vi "Initialize Sim youBot Gripper.vi"(8 "error in (no error)":errorcluster, 10 "arm index":i32, 11 "robot ID":string) -> (0 "error out":errorcluster, 3 "simulated KUKA youBot gripper out":refnum<class "NI_Robotics_KUKA youBot Gripper_Sim.lvclass">)   [LabVIEW 2017, in "NI_Robotics_KUKA youBot Host.lvlib" / "NI_Robotics_KUKA youBot Gripper_Sim.lvclass"]
uses:
  <vilib>/robotics/KUKA youBot/Basic Device/Gripper Sim/NI_Robotics_KUKA youBot Gripper_Sim.lvclass
  c:/Program Files (x86)/National Instruments/LabVIEW 2017/vi.lib/robotics/KUKA youBot/Basic Device/Gripper/NI_Robotics_KUKA youBot Gripper.lvclass
  <vilib>/robotics/Simulator/Engine/ctl/DeviceID.ctl
  <vilib>/robotics/KUKA youBot/Motor/Gripper Motor Sim/NI_Robotics_KUKA youBot Gripper Motor_Sim.lvclass
  c:/Program Files (x86)/National Instruments/LabVIEW 2017/vi.lib/robotics/KUKA youBot/Motor/Gripper Motor/NI_Robotics_KUKA youBot Gripper Motor.lvclass
  <vilib>/robotics/Simulator/NI_Robotics_Simulator.lvlib
  <vilib>/robotics/KUKA youBot/Basic Device/Gripper/NI_Robotics_KUKA youBot Gripper.lvclass
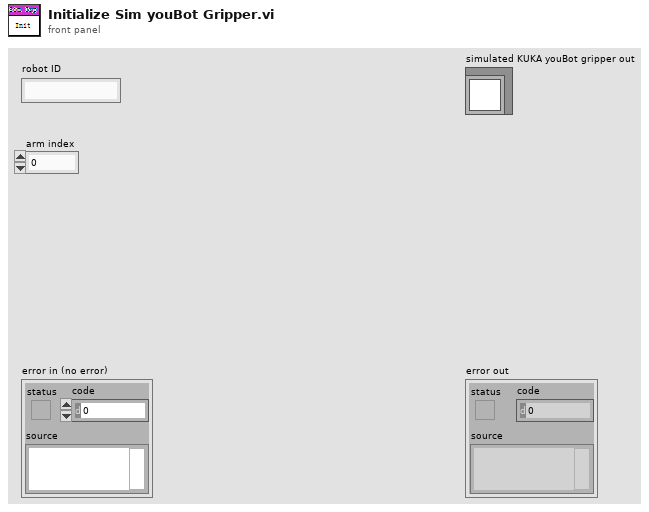
[diagram p1: front panel]
types:
  T1 = typedef "NI_Robotics_Simulator.lvlib/DeviceID.ctl" = cluster{"robot ID":string, "sensor/actuator ID":string}
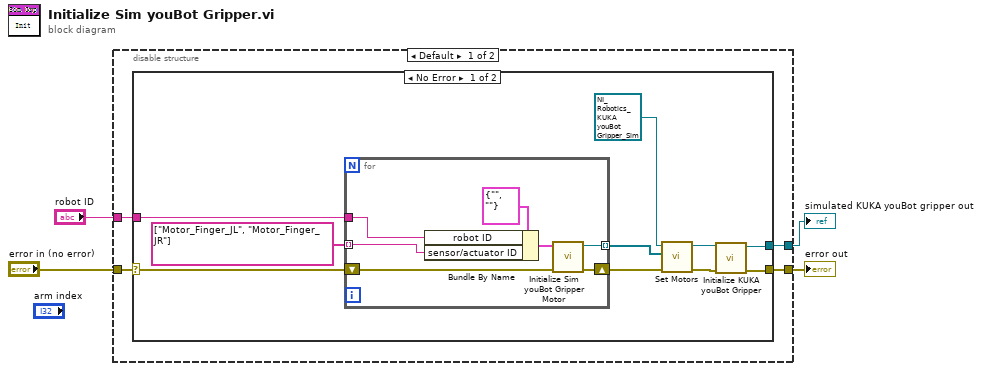
[diagram p0: block diagram]
diagram:
  n1 = disable-structure shown="Default" {
    disable-tunnel: "error in (no error)" -> [w8 _]
    disable-tunnel: [w7 _] -> w3
    disable-tunnel: "robot ID" -> [w6 _]
    disable-tunnel: [w5 _] -> w1
    frame condition #0 (active) {
      n2 = case shown="No Error" w8 {
        selector: w8 -> [w16 w26]
        tunnel: [w10 w26] -> w7
        tunnel: w6 -> [w18 _]
        tunnel: [w9 _] -> w5
        frame No Error {
          n3 = for {
            tunnel: w18 -> [w24]
            tunnel: string[] ["Motor_Finger_JL", "Motor_Finger_JR"] -> [w23] mode=indexing
            shift-right: [w20] -> w14
            shift-left: w16 -> [w21]
            tunnel: [w19] -> w13 mode=indexing
            n4 = Bundle By Name(cluster=T1 {"robot ID"="", "sensor/actuator ID"=""} ("device ID"), "robot ID"=w24, "sensor/actuator ID"=w23) -> (w22:T1)
            n5 = call <vilib>:"Initialize Sim youBot Gripper Motor.vi"("error in (no error)"=w21, "device ID"=w22) -> ("error out"=w20:errorcluster, "simulated KUKA youBot gripper motor out"=w19:refnum<class "NI_Robotics_KUKA youBot Gripper Motor_Sim.lvclass">)  [unwired: 8 in]
          }
          n6 = call-dynamic "Set Motors.vi"("error in (no error)"=w14, "motors"=w13, "KUKA youBot gripper in"=refnum<class "NI_Robotics_KUKA youBot Gripper_Sim.lvclass"> refnum ("NI_Robotics_KUKA youBot Host.lvlib:NI_Robotics_KUKA youBot Gripper_Sim.lvclass")) -> ("error out"=w11:errorcluster, "KUKA youBot gripper out"=w12:refnum<class "NI_Robotics_KUKA youBot Gripper_Sim.lvclass">)  [unwired: 7 in]
          n7 = call <vilib>:"Initialize KUKA youBot Gripper.vi"("error in (no error)"=w11, "KUKA youBot gripper in"=w12) -> ("error out"=w10:errorcluster, "KUKA youBot gripper out"=w9:refnum<class "NI_Robotics_KUKA youBot Gripper_Sim.lvclass">)  [unwired: 8 in]
        }
        frame Error {
        }
      }
    }
    frame condition #1 {
    }
  }
  "error out" <- w3
  "simulated KUKA youBot gripper out" <- w1
